vi "FTW-Test-JobScheduler.vi"() -> (0 "Test Result":errorcluster)   [LabVIEW 2015]
uses:
  src/error/FTW-ERR-ThrowGenericError.vi
  src/error/FTW-ERR-ThrowInfo.vi
  src/error/FTW-ERR-ThrowError.vi
  src/error/FTW-ERR-CallChain.vi
  src/string/FTW-STR-ReplaceWhitespace.vi
  src/string/FTW-STR-Array-Delimit.vi
  src/error/FTW-ERR-Clear.vi
  src/regex/FTW-Regex-ReplaceAll.vi
  src/actor/scheduler/FTW-Scheduler.lvclass
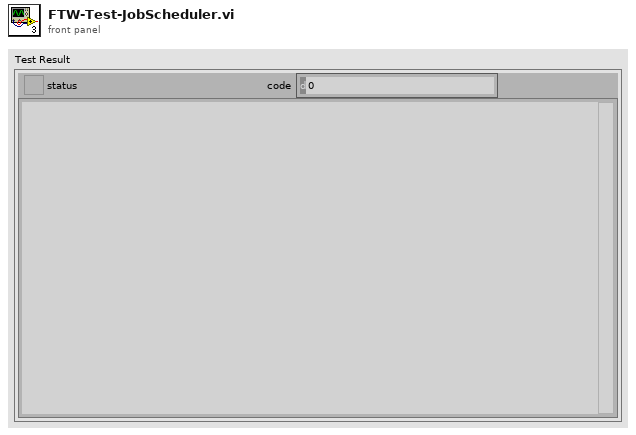
[diagram p1: front panel]
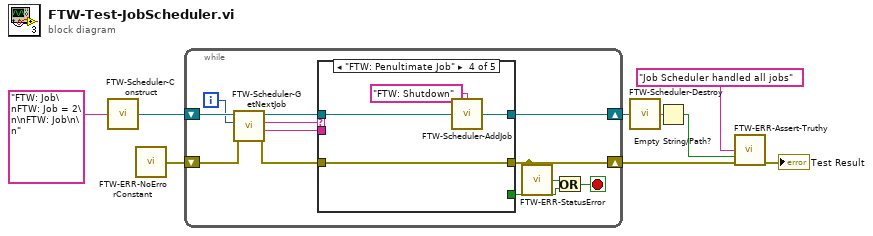
[diagram p0: block diagram]
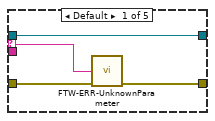
[diagram p2: hidden frame]
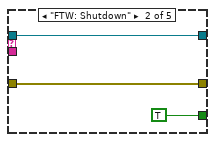
[diagram p3: hidden frame]
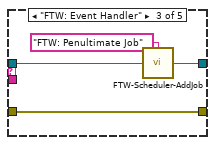
[diagram p4: hidden frame]
diagram:
  n1 = call "FTW-Scheduler-Construct.vi"("Initial Job Sequence"="FTW: Job\nFTW: Job = 2\n\nFTW: Job\n\n") -> ("FTW Job Scheduler"=w9:refnum<class "FTW-Scheduler.lvclass">)
  n2 = call "FTW-ERR-NoErrorConstant.vi"() -> ("no error"=w6:errorcluster)
  n3 = while {
    shift-right: [w12] -> w7
    shift-left: w9 -> [w21]
    shift-right: [w15] -> w4
    shift-left: w6 -> [w20]
    i -> [w19]
    stop <- w13 stop-if-true
    n4 = call "FTW-Scheduler-GetNextJob.vi"("error in"=w20, "Jobs Performed"=w19, "FTW Job Scheduler"=w21) -> ("error out"=w16:errorcluster, "Job Data"=w11:string, "Current Job"=w18:string, "FTW Job Scheduler out"=w10:refnum<class "FTW-Scheduler.lvclass">)  [unwired: 5 in]
    n5 = case shown="\"FTW: Penultimate Job\"" w18 {
      selector: w18 -> [w24 _ _ _ _]
      tunnel: w10 -> [w25 w26 w31 w35 w37]
      tunnel: [_ TRUE _ _ _] -> w14
      tunnel: w16 -> [w23 w27 w32 w36 w38]
      tunnel: [w22 w27 w32 w36 w38] -> w15
      tunnel: [w25 w26 w30 w34 w37] -> w12
      tunnel: w11 -> [_ _ _ _ _]
      frame Default {
        n6 = call "FTW-ERR-UnknownParameter.vi"("Unknown Parameter"=w24, "error in"=w23) -> ("error out"=w22:errorcluster)  [unwired: 13 in]
      }
      frame "FTW: Shutdown" {
      }
      frame "FTW: Event Handler" {
        n7 = call "FTW-Scheduler-AddJob.vi"("Add to Job Sequence"="FTW: Penultimate Job" ("Add Next in Sequence"), "FTW Job Scheduler"=w31) -> ("FTW Job Scheduler out"=w30:refnum<class "FTW-Scheduler.lvclass">)  [unwired: 2 in]
      }
      frame "FTW: Penultimate Job" {
        n8 = call "FTW-Scheduler-AddJob.vi"("Add to Job Sequence"="FTW: Shutdown" ("Add Next in Sequence"), "FTW Job Scheduler"=w35) -> ("FTW Job Scheduler out"=w34:refnum<class "FTW-Scheduler.lvclass">)  [unwired: 2 in]
      }
      frame "FTW: Job" {
      }
    }
    n9 = call "FTW-ERR-StatusError.vi"("error to check"=w15) -> ("Error?"=w17:bool)
    n10 = Or(x=w17, y=w14) -> (x .or. y?=w13:bool)
  }
  n11 = call "FTW-Scheduler-Destroy.vi"("FTW Job Scheduler"=w7) -> ("Remaining Jobs"=w5:string)
  n12 = Empty String/Path?(string/path=w5) -> (empty?=w2:bool)
  n13 = call "FTW-ERR-Assert-Truthy.vi"("Assertion"="Job Scheduler handled all jobs", "Assertion holds true?"=w2, "error in"=w4) -> ("error out"=→"Test Result":errorcluster)  [unwired: 12 in]
